vi "Append VI Block Diagram to Report.vi"   [LabVIEW 2017, in "NI_ReportGenerationCore.lvlib"]
doc: "Creates an image of the block diagram of the VI you specify in <B>VI</B> and appends the image to a report. Wire data to the <B>VI</B> input to determine the polymorphic instance to use or manually select the instance."
uses:
  <vilib>/Utility/NIReport.llb/NI_ReportGenerationCore.lvlib
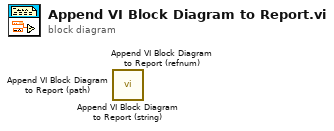
[diagram p0: block diagram]
diagram:
  n1 = call <vilib>:"Append VI Block Diagram to Report (string).vi"() -> ()  [unwired: 11 in, 5 out]
  n2 = call <vilib>:"Append VI Block Diagram to Report (refnum).vi"() -> ()  [unwired: 11 in, 5 out]
  n3 = call <vilib>:"Append VI Block Diagram to Report (path).vi"() -> ()  [unwired: 11 in, 5 out]
